vi "Time Until Next.vi"(8 "error in (no error)":errorcluster, 11 "ARecurrence in":refnum<class "ARecurrence.lvclass">) -> (0 "error out":errorcluster, 1 "Time Stamp of Next":timestamp, 2 "Seconds Until Next Tick":u32, 3 "ARecurrence out":refnum<class "ARecurrence.lvclass">)   [LabVIEW 2020, in "ARecurrence.lvclass"]
uses:
  ARecurrence.lvclass
  ARecurrence.lvclass/ARecurrence.ctl
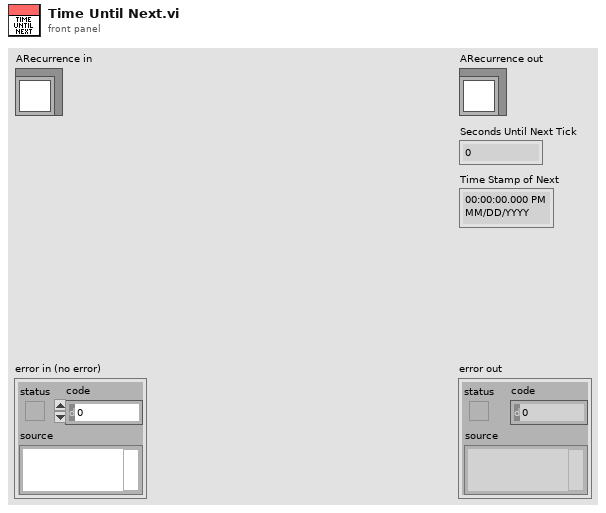
[diagram p1: front panel]
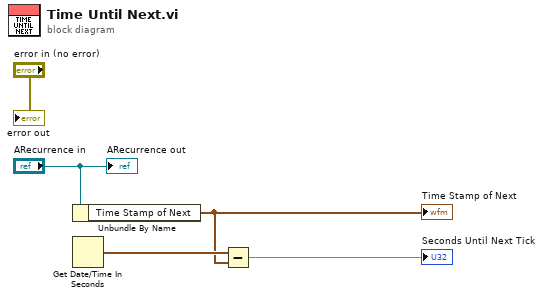
[diagram p0: block diagram]
diagram:
  n1 = Unbundle By Name("ARecurrence in") -> ("Time Stamp of Next"=w2:timestamp)
  "Time Stamp of Next" <- w2
  n2 = Get Date/Time In Seconds() -> (seconds since 1Jan1904=w3:timestamp)
  n3 = Subtract(x=w3, y=w2) -> (x-y=→"Seconds Until Next Tick":dbl)
  "error out" <- "error in (no error)"
  "ARecurrence out" <- "ARecurrence in"
